vi "Edit Filter and Sort Options.vi"() -> ()   [LabVIEW 2023, in "VI Properties Editor.lvlib"]
uses:
  VI Properties Editor.lvlib
panel:
  in  "Filter Value":string
  in  "Filter Type":enum16{""}(ring)
  in  "Sort Order":enum16{""}(ring)
  in  "Sort Column":enum16{""}(ring)
  in  "Filter Column":enum16{""}(ring)
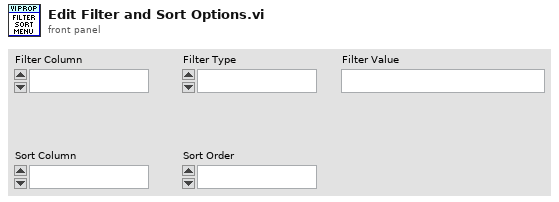
[diagram p1: front panel]
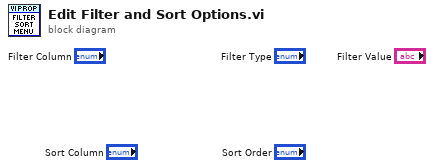
[diagram p0: block diagram]
diagram:
